vi "veristandSteps-installer-update.vi"   [LabVIEW 2014, in "veristand-steps-build-system.lvlib"]
uses:
  veristand-steps-build-system.lvlib
  <vilib>/Wiresmith Technology/LabVIEW CLI/CLI Class/CLI.lvclass
types:
  T1 = typedef "lv-build-library.lvlib/LVInstallerMutationSession.ctl" = cluster{"Installer Build Specification Ref":refnum<vi>, "Project reference out":refnum<vi>, "Installer Project Path":path}
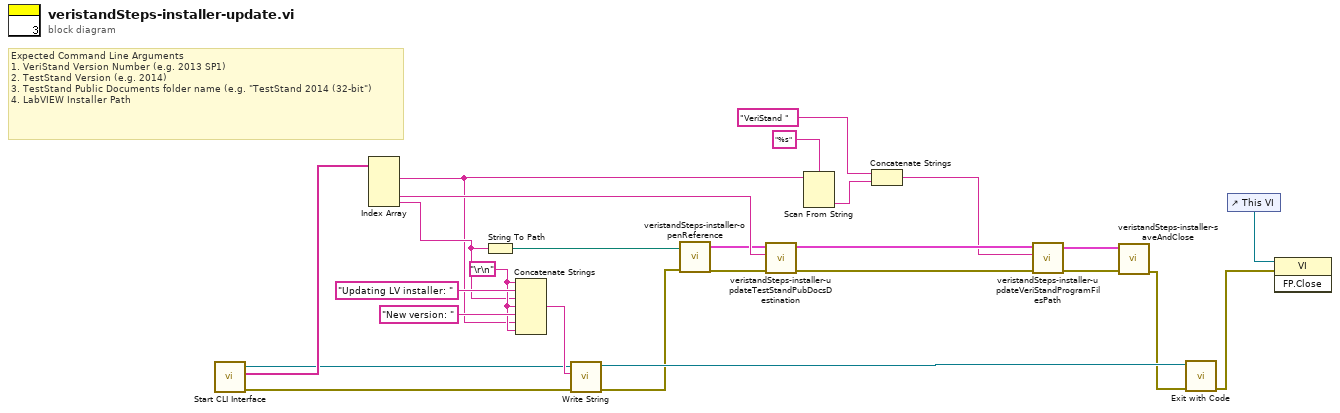
[diagram p0: block diagram]
diagram:
  w20 = "\r\n"
  # "Expected Command Line Arguments\n1. VeriStand Version Number (e.g. 2013 SP1)\n2. TestStand Version (e.g. 2014)\n3. TestStand Public Documents folder name (e.g. \"TestStand 2014 (32-bit\")\n4. LabVIEW Installer Path"
  n1 = call <vilib>:"Start CLI Interface.vi"() -> ("error out"=w23:errorcluster, "Custom Parameters"=w24:string[], "CLI out"=w18:refnum<class "CLI.lvclass">)  [unwired: 9 in]
  n2 = Index Array(array=w24) -> (element #1=w3:string, element #3=w4:string, element #4=w5:string)  [unwired: 4 in, 1 out]
  n3 = String To Path(string=w5) -> (path=w25:path)
  n4 = Concatenate Strings(w20, "Updating LV installer: " ("string"), w5, w20, "New version: " ("string"), w3, w20) -> (w19:string)
  n5 = call <vilib>:"Write String.vi"("error in (no error)"=w23, "Text to Write"=w19, "CLI in"=w18) -> ("error out"=w15:errorcluster, "CLI out"=w16:refnum<class "CLI.lvclass">)  [unwired: 7 in]
  n6 = call "veristandSteps-installer-openReference.vi"("error in (no error)"=w15, "Installer Project Path"=w25) -> ("error out"=w1:errorcluster, "InstallerSession"=w2:T1)  [unwired: 8 in]
  n7 = call "veristandSteps-installer-updateTestStandPubDocsDestination.vi"("error in (no error)"=w1, "TestStand Public Docs Folder Name"=w4, "InstallerMutationSession"=w2) -> ("error out"=w13:errorcluster, "InstallerMutationSession out"=w7:T1)  [unwired: 7 in]
  n8 = Scan From String(format string="%s", input string=w3) -> (output 1=w8:string)  [unwired: 3 in, 3 out]
  n9 = Concatenate Strings("VeriStand " ("string"), w8) -> (w6:string)
  n10 = call "veristandSteps-installer-updateVeriStandProgramFilesPath.vi"("error in (no error)"=w13, "VeriStand Applicatin Program Files Directroy"=w6, "InstallerMutationSession"=w7) -> ("error out"=w12:errorcluster, "InstallerMutationSession out"=w11:T1)  [unwired: 7 in]
  n11 = call "veristandSteps-installer-saveAndClose.vi"("error in (no error)"=w12, "InstallerMutationSession"=w11) -> ("error out"=w14:errorcluster)  [unwired: 9 in]
  n12 = call <vilib>:"Exit with Code.vi"("error in (no error)"=w14, "CLI in"=w16) -> ("error out"=w17:errorcluster)  [unwired: 9 in]
  n13 = control-ref of="This VI"() -> (w26:refnum<vi>)
  n14 = invoke class="VI" method="FP.Close"(reference=w26, error in=w17) -> ()  [unwired: 1 in, 3 out]
